vi "LoadTileSheet.vi"(8 "error in (no error)":errorcluster, 10 "Tile Path":path, 11 "Game in":refnum<class "Game.lvclass">) -> (0 "error out":errorcluster, 3 "Game out":refnum<class "Game.lvclass">)   [LabVIEW 2019, in "RT_Game.lvlib" / "Game.lvclass"]
uses:
  Game.lvclass
  Game.lvclass/Game.ctl
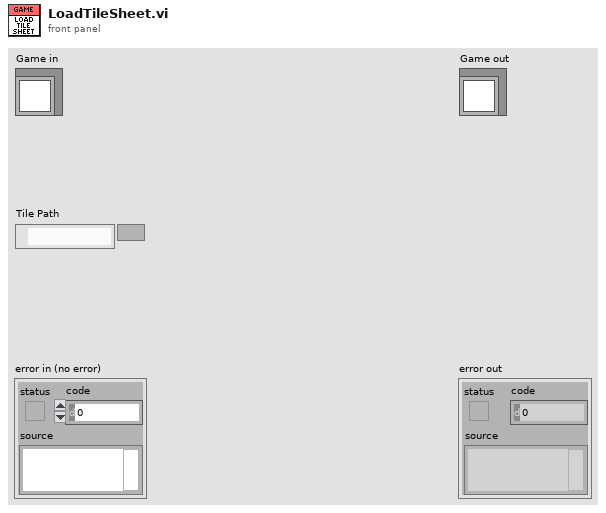
[diagram p1: front panel]
types:
  T1 = typedef "FPGA_Interface.ctl" = refnum<k20>
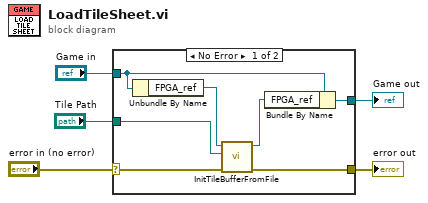
[diagram p0: block diagram]
diagram:
  n1 = case shown="No Error" "error in (no error)" {
    selector: "error in (no error)" -> [w12 w14]
    tunnel: [w10 w14] -> w4
    tunnel: [w9 w13] -> w2
    tunnel: "Game in" -> [w11 w13]
    tunnel: "Tile Path" -> [w7 _]
    frame No Error {
      n2 = Unbundle By Name(w11) -> ("FPGA_ref"=w6:T1)
      n3 = call "InitTileBufferFromFile.vi"("error in (no error)"=w12, "Tile Path"=w7, "Refnum in"=w6) -> ("error out"=w10:errorcluster, "Refnum out"=w8:T1)  [unwired: 7 in]
      n4 = Bundle By Name(cluster=w11, "FPGA_ref"=w8) -> (w9:refnum<class "Game.lvclass">)
    }
    frame Error {
    }
  }
  "error out" <- w4
  "Game out" <- w2
